vi "数据发送组合-20200825 (子VI).vi"(10 "枚举":T2(ring), 11 "插值后的数组元素":T1) -> (3 "字符串":string)   [LabVIEW 2016, in "数据传输系统-02.lvlib"]
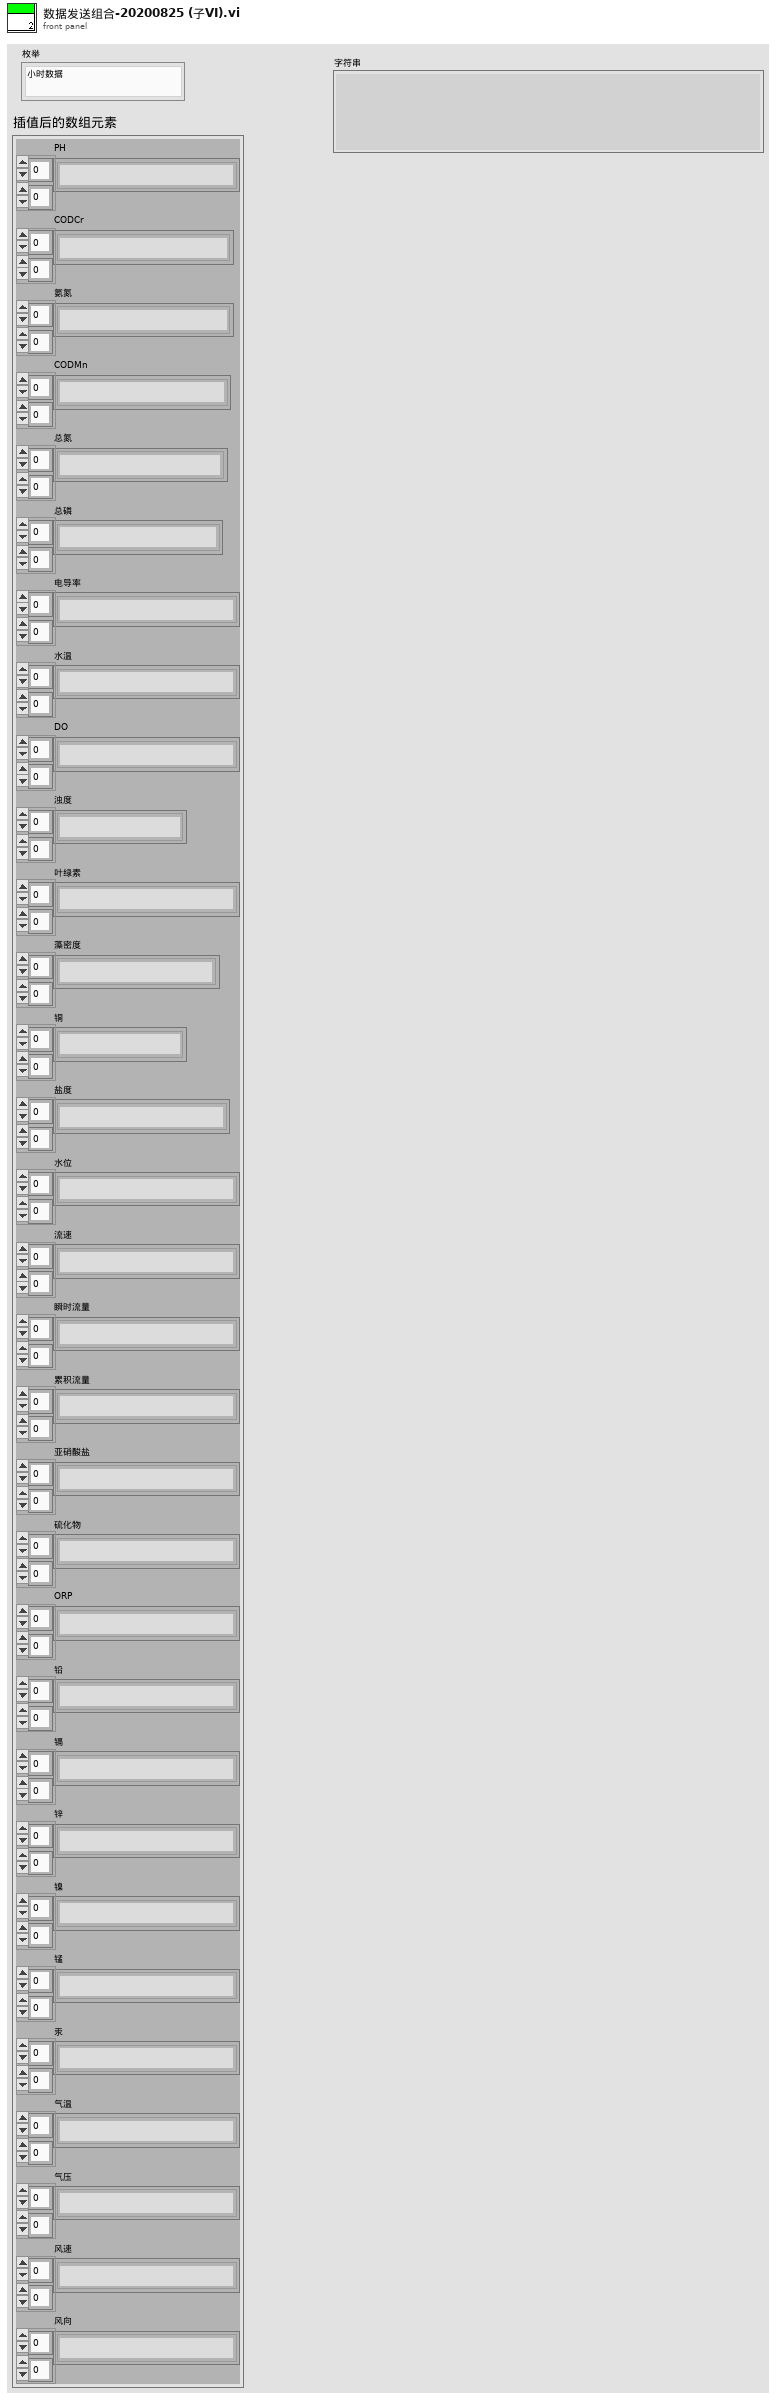
[diagram p1: front panel]
types:
  T1 = cluster{"PH":string[][], "CODCr":string[][], "氨氮":string[][], "CODMn":string[][], "总氮":string[][], "总磷":string[][], "电导率":string[][], "水温":string[][], "DO":string[][], "浊度":string[][], "叶绿素":string[][], "藻密度":string[][], "铜":string[][], "盐度":string[][], "水位":string[][], "流速":string[][], "瞬时流量":string[][], "累积流量":string[][], "亚硝酸盐":string[][], "硫化物":string[][], "ORP":string[][], "铅":string[][], "镉":string[][], "锌":string[][], "镍":string[][], "锰":string[][], "汞":string[][], "气温":string[][], "气压":string[][], "风速":string[][], "风向":string[][]}
  T2 = enum16{"小时数据", "实时数据", "平行样测试", "集成干预测试", "加标回收测试", "核查数据", "空白零点跨度数据", "提取小时数据", "提取实时数据", "操作日志", "仪器参数", "3090仪器参数", "提取仪器参数", "报警信息"}
  T3 = cluster{"CODMn":string, "CODCr":string, "DO":string, "铜":string, "PH":string, "氨氮":string, "比电导率":string, "水温":string, "COD":string, "浊度":string, "总氮":string, "总磷":string, "叶绿素a":string, "藻密度":string, "水位":string, "流速":string, "瞬时流量":string, "累积流量":string, "亚硝酸盐":string, "硫化物":string, "ORP":string, "铅":string, "镉":string, "锌":string, "镍":string, "锰":string, "汞":string, "气温":string, "气压":string, "风速":string, "风向":string}
  T4 = cluster{"CODMn":dbl, "CODCr":dbl, "DO":dbl, "铜":dbl, "PH":dbl, "氨氮":dbl, "比电导率":dbl, "水温":dbl, "COD":dbl, "浊度":dbl, "总氮":dbl, "总磷":dbl, "叶绿素a":dbl, "藻密度":dbl, "水位":dbl, "流速":dbl, "瞬时流量":dbl, "累积流量":dbl, "亚硝酸盐":dbl, "硫化物":dbl, "ORP":dbl, "铅":dbl, "镉":dbl, "锌":dbl, "镍":dbl, "锰":dbl, "汞":dbl, "气温":dbl, "气压":dbl, "风速":dbl, "风向":dbl}
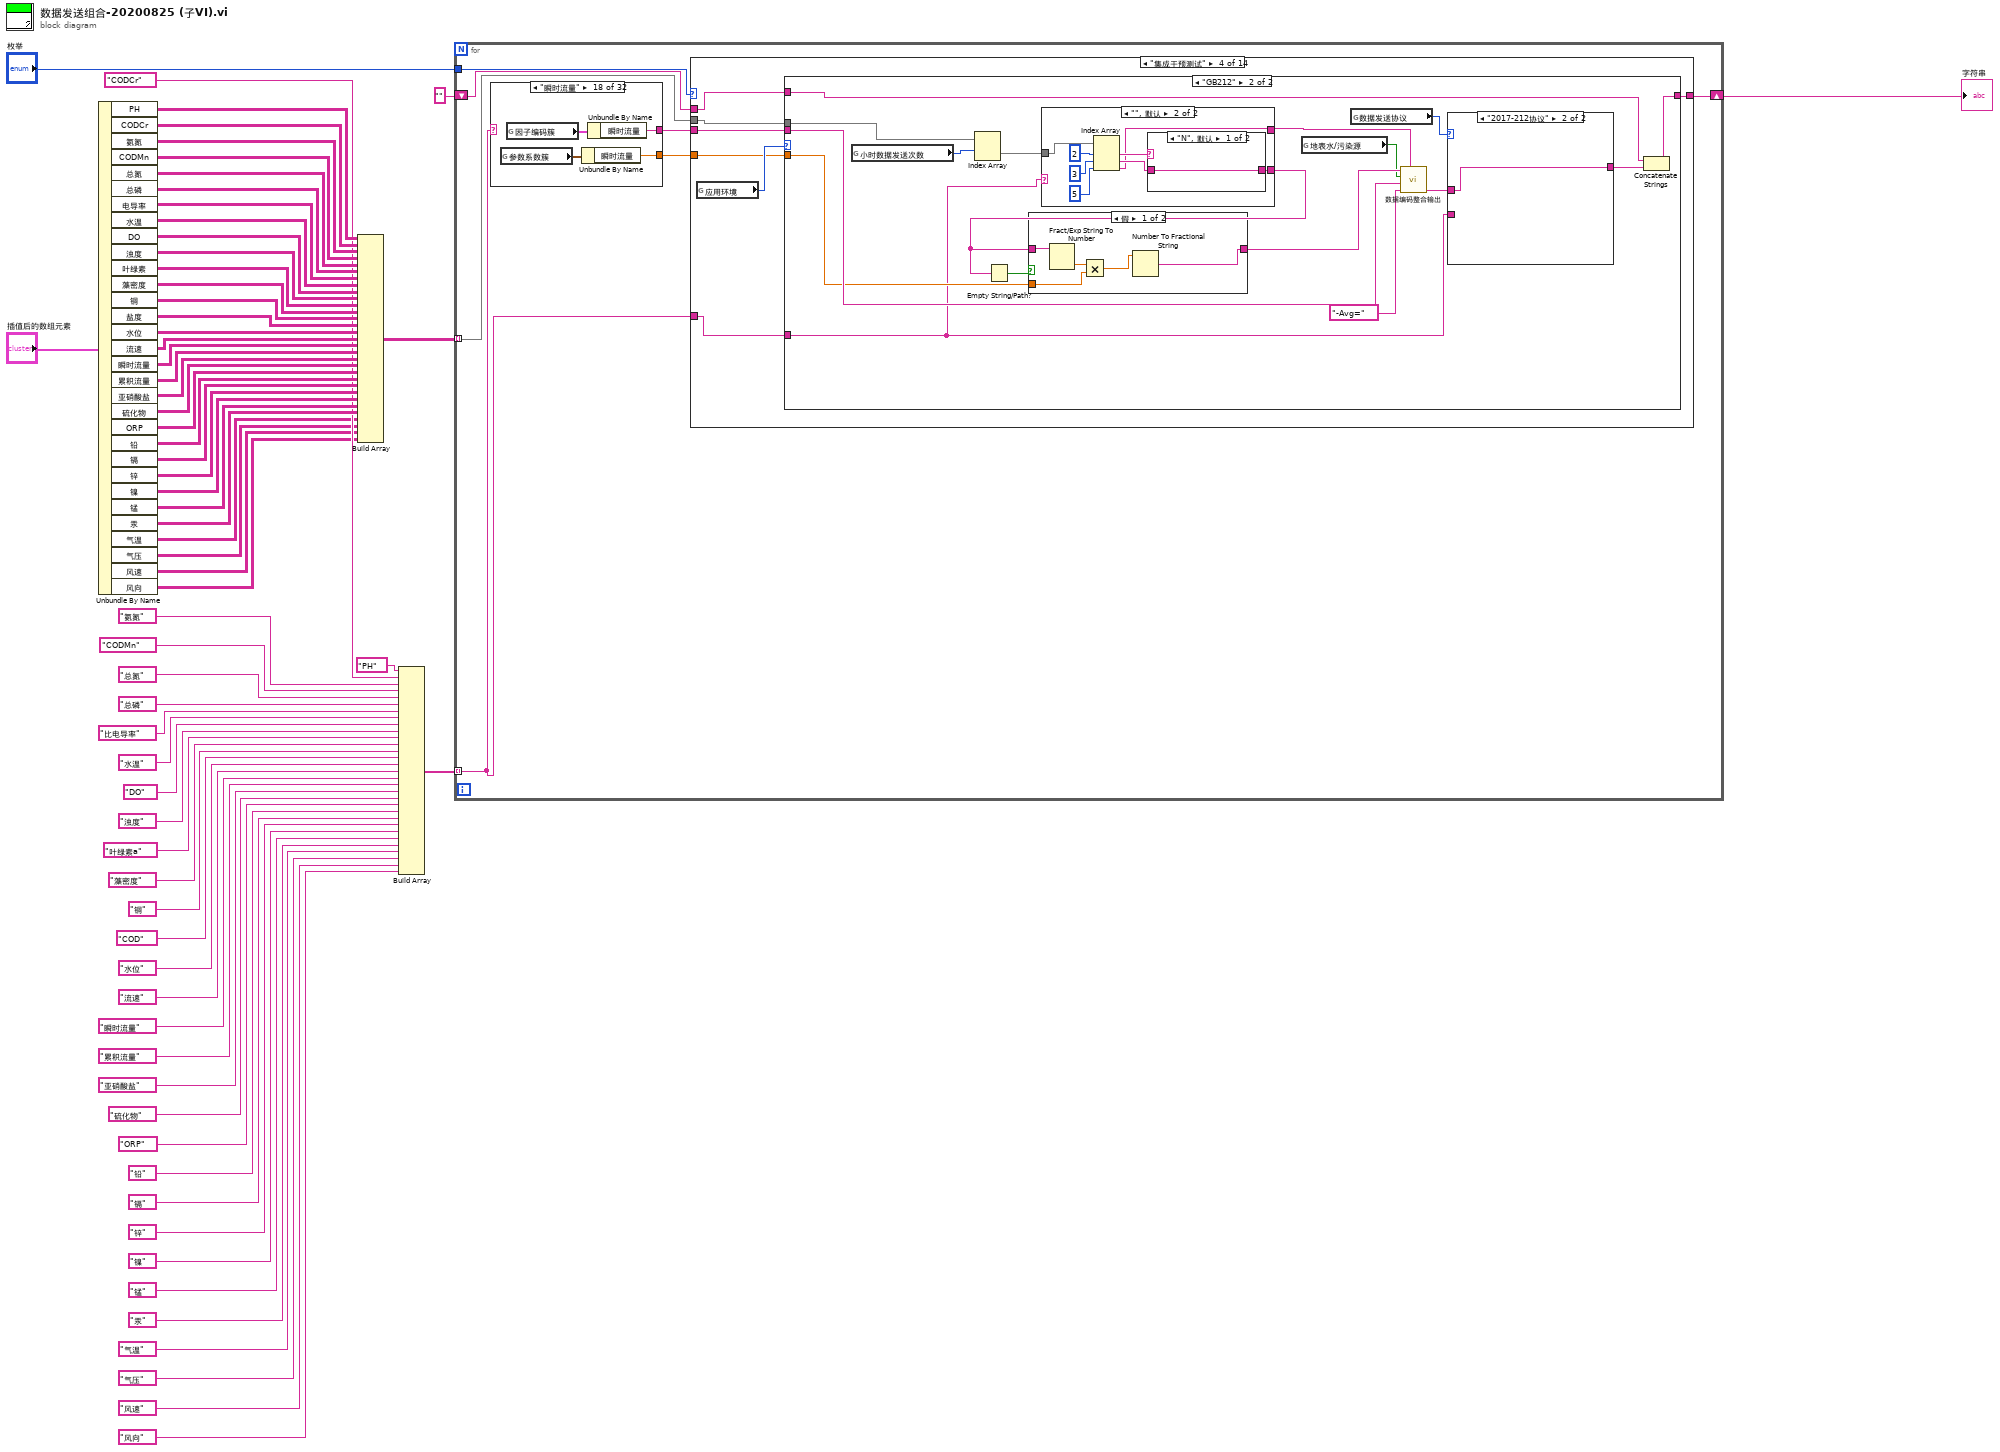
[diagram p0: block diagram]
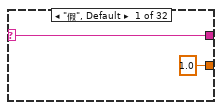
[diagram p2: hidden frame]
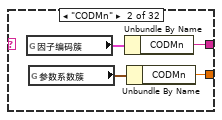
[diagram p3: hidden frame]
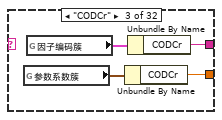
[diagram p4: hidden frame]
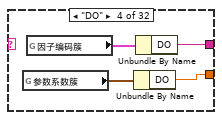
[diagram p5: hidden frame]
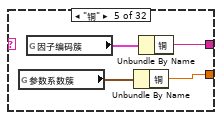
[diagram p6: hidden frame]
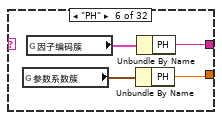
[diagram p7: hidden frame]
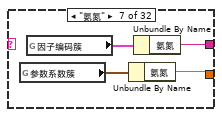
[diagram p8: hidden frame]
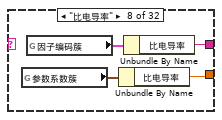
[diagram p9: hidden frame]
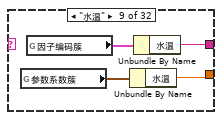
[diagram p10: hidden frame]
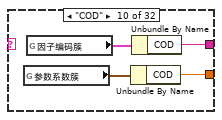
[diagram p11: hidden frame]
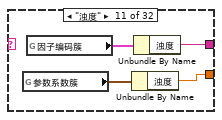
[diagram p12: hidden frame]
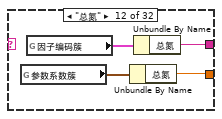
[diagram p13: hidden frame]
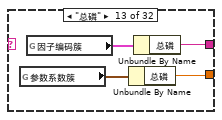
[diagram p14: hidden frame]
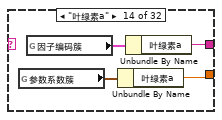
[diagram p15: hidden frame]
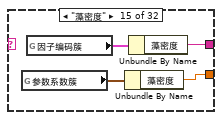
[diagram p16: hidden frame]
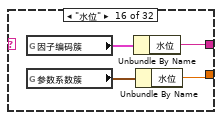
[diagram p17: hidden frame]
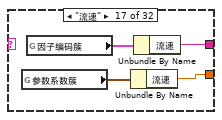
[diagram p18: hidden frame]
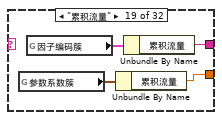
[diagram p19: hidden frame]
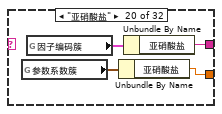
[diagram p20: hidden frame]
diagram:
  n1 = Unbundle By Name("插值后的数组元素") -> ("PH"=w68:string[][], "CODCr"=w67:string[][], "氨氮"=w66:string[][], "CODMn"=w65:string[][], "总氮"=w64:string[][], "总磷"=w63:string[][], "电导率"=w62:string[][], "水温"=w61:string[][], "DO"=w60:string[][], "浊度"=w59:string[][], "叶绿素"=w58:string[][], "藻密度"=w57:string[][], "铜"=w56:string[][], "盐度"=w55:string[][], "水位"=w54:string[][], "流速"=w53:string[][], "瞬时流量"=w52:string[][], "累积流量"=w51:string[][], "亚硝酸盐"=w50:string[][], "硫化物"=w49:string[][], "ORP"=w48:string[][], "铅"=w47:string[][], "镉"=w46:string[][], "锌"=w45:string[][], "镍"=w44:string[][], "锰"=w43:string[][], "汞"=w42:string[][], "气温"=w5:string[][], "气压"=w6:string[][], "风速"=w7:string[][], "风向"=w8:string[][])
  n2 = Build Array(w68, w67, w66, w65, w64, w63, w62, w61, w60, w59, w58, w57, w56, w55, w54, w53, w52, w51, w50, w49, w48, w47, w46, w45, w44, w43, w42, w5, w6, w7, w8) -> (w41:string[][][])
  n3 = Build Array("PH" ("污染物编码"), "CODCr" ("污染物编码"), "氨氮" ("污染物编码"), "CODMn" ("污染物编码"), "总氮" ("污染物编码"), "总磷" ("污染物编码"), "比电导率" ("污染物编码"), "水温" ("污染物编码"), "DO" ("污染物编码"), "浊度" ("污染物编码"), "叶绿素a" ("污染物编码"), "藻密度" ("污染物编码"), "铜" ("污染物编码"), "COD" ("污染物编码"), "水位" ("污染物编码"), "流速" ("污染物编码"), "瞬时流量" ("污染物编码"), "累积流量" ("污染物编码"), "亚硝酸盐" ("污染物编码"), "硫化物" ("污染物编码"), "ORP" ("污染物编码"), "铅" ("污染物编码"), "镉" ("污染物编码"), "锌" ("污染物编码"), "镍" ("污染物编码"), "锰" ("污染物编码"), "汞" ("污染物编码"), "气温" ("污染物编码"), "气压" ("污染物编码"), "风速" ("污染物编码"), "风向" ("污染物编码")) -> (w13:string[])
  n4 = for {
    tunnel: w41 -> [w75] mode=indexing
    tunnel: w13 -> [w70] mode=indexing
    shift-right: [w74] -> w11
    shift-left: "" -> [w73]
    tunnel: "枚举" -> [w72]
    n5 = case shown="\"瞬时流量\"" w70 {
      selector: w70 -> [w77 _ _ _ _ _ _ _ _ _ _ _ _ _ _ _ _ _ _ _ _ _ _ _ _ _ _ _ _ _ _ _]
      tunnel: [w77 w80 w84 w88 w92 w96 w100 w104 w108 w112 w116 w120 w124 w128 w132 w136 w140 w144 w148 w152 w156 w160 w164 w168 w172 w176 w180 w184 w188 w192 w196 w200] -> w71
      tunnel: [1.0 ("风向") w78 w82 w86 w90 w94 w98 w102 w106 w110 w114 w118 w122 w126 w130 w134 w138 w142 w146 w150 w154 w158 w162 w166 w170 w174 w178 w182 w186 w190 w194 w198] -> w69
      frame "假", Default {
      }
      frame "CODMn" {
        n6 = global read "断电保存全局.vi" "因子编码簇"() -> (w81:T3)
        n7 = global read "断电保存全局.vi" "参数系数簇"() -> (w79:T4)
        n8 = Unbundle By Name(w81) -> ("CODMn"=w80:string)
        n9 = Unbundle By Name(w79) -> ("CODMn"=w78:dbl)
      }
      frame "CODCr" {
        n10 = global read "断电保存全局.vi" "参数系数簇"() -> (w83:T4)
        n11 = global read "断电保存全局.vi" "因子编码簇"() -> (w85:T3)
        n12 = Unbundle By Name(w83) -> ("CODCr"=w82:dbl)
        n13 = Unbundle By Name(w85) -> ("CODCr"=w84:string)
      }
      frame "DO" {
        n14 = global read "断电保存全局.vi" "参数系数簇"() -> (w87:T4)
        n15 = global read "断电保存全局.vi" "因子编码簇"() -> (w89:T3)
        n16 = Unbundle By Name(w87) -> ("DO"=w86:dbl)
        n17 = Unbundle By Name(w89) -> ("DO"=w88:string)
      }
      frame "铜" {
        n18 = global read "断电保存全局.vi" "参数系数簇"() -> (w91:T4)
        n19 = global read "断电保存全局.vi" "因子编码簇"() -> (w93:T3)
        n20 = Unbundle By Name(w91) -> ("铜"=w90:dbl)
        n21 = Unbundle By Name(w93) -> ("铜"=w92:string)
      }
      frame "PH" {
        n22 = global read "断电保存全局.vi" "参数系数簇"() -> (w95:T4)
        n23 = global read "断电保存全局.vi" "因子编码簇"() -> (w97:T3)
        n24 = Unbundle By Name(w95) -> ("PH"=w94:dbl)
        n25 = Unbundle By Name(w97) -> ("PH"=w96:string)
      }
      frame "氨氮" {
        n26 = global read "断电保存全局.vi" "参数系数簇"() -> (w99:T4)
        n27 = global read "断电保存全局.vi" "因子编码簇"() -> (w101:T3)
        n28 = Unbundle By Name(w99) -> ("氨氮"=w98:dbl)
        n29 = Unbundle By Name(w101) -> ("氨氮"=w100:string)
      }
      frame "比电导率" {
        n30 = global read "断电保存全局.vi" "参数系数簇"() -> (w103:T4)
        n31 = global read "断电保存全局.vi" "因子编码簇"() -> (w105:T3)
        n32 = Unbundle By Name(w103) -> ("比电导率"=w102:dbl)
        n33 = Unbundle By Name(w105) -> ("比电导率"=w104:string)
      }
      frame "水温" {
        n34 = global read "断电保存全局.vi" "参数系数簇"() -> (w107:T4)
        n35 = global read "断电保存全局.vi" "因子编码簇"() -> (w109:T3)
        n36 = Unbundle By Name(w107) -> ("水温"=w106:dbl)
        n37 = Unbundle By Name(w109) -> ("水温"=w108:string)
      }
      frame "COD" {
        n38 = global read "断电保存全局.vi" "参数系数簇"() -> (w111:T4)
        n39 = global read "断电保存全局.vi" "因子编码簇"() -> (w113:T3)
        n40 = Unbundle By Name(w111) -> ("COD"=w110:dbl)
        n41 = Unbundle By Name(w113) -> ("COD"=w112:string)
      }
      frame "浊度" {
        n42 = global read "断电保存全局.vi" "参数系数簇"() -> (w115:T4)
        n43 = global read "断电保存全局.vi" "因子编码簇"() -> (w117:T3)
        n44 = Unbundle By Name(w115) -> ("浊度"=w114:dbl)
        n45 = Unbundle By Name(w117) -> ("浊度"=w116:string)
      }
      frame "总氮" {
        n46 = global read "断电保存全局.vi" "参数系数簇"() -> (w119:T4)
        n47 = global read "断电保存全局.vi" "因子编码簇"() -> (w121:T3)
        n48 = Unbundle By Name(w119) -> ("总氮"=w118:dbl)
        n49 = Unbundle By Name(w121) -> ("总氮"=w120:string)
      }
      frame "总磷" {
        n50 = global read "断电保存全局.vi" "参数系数簇"() -> (w123:T4)
        n51 = global read "断电保存全局.vi" "因子编码簇"() -> (w125:T3)
        n52 = Unbundle By Name(w123) -> ("总磷"=w122:dbl)
        n53 = Unbundle By Name(w125) -> ("总磷"=w124:string)
      }
      frame "叶绿素a" {
        n54 = global read "断电保存全局.vi" "参数系数簇"() -> (w127:T4)
        n55 = global read "断电保存全局.vi" "因子编码簇"() -> (w129:T3)
        n56 = Unbundle By Name(w127) -> ("叶绿素a"=w126:dbl)
        n57 = Unbundle By Name(w129) -> ("叶绿素a"=w128:string)
      }
      frame "藻密度" {
        n58 = global read "断电保存全局.vi" "参数系数簇"() -> (w131:T4)
        n59 = global read "断电保存全局.vi" "因子编码簇"() -> (w133:T3)
        n60 = Unbundle By Name(w131) -> ("藻密度"=w130:dbl)
        n61 = Unbundle By Name(w133) -> ("藻密度"=w132:string)
      }
      frame "水位" {
        n62 = global read "断电保存全局.vi" "因子编码簇"() -> (w137:T3)
        n63 = global read "断电保存全局.vi" "参数系数簇"() -> (w135:T4)
        n64 = Unbundle By Name(w137) -> ("水位"=w136:string)
        n65 = Unbundle By Name(w135) -> ("水位"=w134:dbl)
      }
      frame "流速" {
        n66 = global read "断电保存全局.vi" "参数系数簇"() -> (w139:T4)
        n67 = global read "断电保存全局.vi" "因子编码簇"() -> (w141:T3)
        n68 = Unbundle By Name(w139) -> ("流速"=w138:dbl)
        n69 = Unbundle By Name(w141) -> ("流速"=w140:string)
      }
      frame "瞬时流量" {
        n70 = global read "断电保存全局.vi" "参数系数簇"() -> (w143:T4)
        n71 = global read "断电保存全局.vi" "因子编码簇"() -> (w145:T3)
        n72 = Unbundle By Name(w143) -> ("瞬时流量"=w142:dbl)
        n73 = Unbundle By Name(w145) -> ("瞬时流量"=w144:string)
      }
      frame "累积流量" {
        n74 = global read "断电保存全局.vi" "参数系数簇"() -> (w147:T4)
        n75 = global read "断电保存全局.vi" "因子编码簇"() -> (w149:T3)
        n76 = Unbundle By Name(w147) -> ("累积流量"=w146:dbl)
        n77 = Unbundle By Name(w149) -> ("累积流量"=w148:string)
      }
      frame "亚硝酸盐" {
        n78 = global read "断电保存全局.vi" "参数系数簇"() -> (w151:T4)
        n79 = global read "断电保存全局.vi" "因子编码簇"() -> (w153:T3)
        n80 = Unbundle By Name(w151) -> ("亚硝酸盐"=w150:dbl)
        n81 = Unbundle By Name(w153) -> ("亚硝酸盐"=w152:string)
      }
      frame "硫化物" {
        n82 = global read "断电保存全局.vi" "参数系数簇"() -> (w155:T4)
        n83 = global read "断电保存全局.vi" "因子编码簇"() -> (w157:T3)
        n84 = Unbundle By Name(w155) -> ("硫化物"=w154:dbl)
        n85 = Unbundle By Name(w157) -> ("硫化物"=w156:string)
      }
      frame "ORP" {
        n86 = global read "断电保存全局.vi" "参数系数簇"() -> (w159:T4)
        n87 = global read "断电保存全局.vi" "因子编码簇"() -> (w161:T3)
        n88 = Unbundle By Name(w159) -> ("ORP"=w158:dbl)
        n89 = Unbundle By Name(w161) -> ("ORP"=w160:string)
      }
      frame "铅" {
        n90 = global read "断电保存全局.vi" "参数系数簇"() -> (w163:T4)
        n91 = global read "断电保存全局.vi" "因子编码簇"() -> (w165:T3)
        n92 = Unbundle By Name(w165) -> ("铅"=w164:string)
        n93 = Unbundle By Name(w163) -> ("铅"=w162:dbl)
      }
      frame "镉" {
        n94 = global read "断电保存全局.vi" "参数系数簇"() -> (w167:T4)
        n95 = global read "断电保存全局.vi" "因子编码簇"() -> (w169:T3)
        n96 = Unbundle By Name(w167) -> ("镉"=w166:dbl)
        n97 = Unbundle By Name(w169) -> ("镉"=w168:string)
      }
      frame "锌" {
        n98 = global read "断电保存全局.vi" "参数系数簇"() -> (w171:T4)
        n99 = global read "断电保存全局.vi" "因子编码簇"() -> (w173:T3)
        n100 = Unbundle By Name(w171) -> ("锌"=w170:dbl)
        n101 = Unbundle By Name(w173) -> ("锌"=w172:string)
      }
      frame "镍" {
        n102 = global read "断电保存全局.vi" "参数系数簇"() -> (w175:T4)
        n103 = global read "断电保存全局.vi" "因子编码簇"() -> (w177:T3)
        n104 = Unbundle By Name(w175) -> ("镍"=w174:dbl)
        n105 = Unbundle By Name(w177) -> ("镍"=w176:string)
      }
      frame "锰" {
        n106 = global read "断电保存全局.vi" "参数系数簇"() -> (w179:T4)
        n107 = global read "断电保存全局.vi" "因子编码簇"() -> (w181:T3)
        n108 = Unbundle By Name(w181) -> ("锰"=w180:string)
        n109 = Unbundle By Name(w179) -> ("锰"=w178:dbl)
      }
      frame "汞" {
        n110 = global read "断电保存全局.vi" "参数系数簇"() -> (w183:T4)
        n111 = global read "断电保存全局.vi" "因子编码簇"() -> (w185:T3)
        n112 = Unbundle By Name(w185) -> ("汞"=w184:string)
        n113 = Unbundle By Name(w183) -> ("汞"=w182:dbl)
      }
      frame "气温" {
        n114 = global read "断电保存全局.vi" "因子编码簇"() -> (w189:T3)
        n115 = global read "断电保存全局.vi" "参数系数簇"() -> (w187:T4)
        n116 = Unbundle By Name(w189) -> ("气温"=w188:string)
        n117 = Unbundle By Name(w187) -> ("气温"=w186:dbl)
      }
      frame "气压" {
        n118 = global read "断电保存全局.vi" "参数系数簇"() -> (w191:T4)
        n119 = global read "断电保存全局.vi" "因子编码簇"() -> (w193:T3)
        n120 = Unbundle By Name(w191) -> ("气压"=w190:dbl)
        n121 = Unbundle By Name(w193) -> ("气压"=w192:string)
      }
      frame "风速" {
        n122 = global read "断电保存全局.vi" "参数系数簇"() -> (w195:T4)
        n123 = global read "断电保存全局.vi" "因子编码簇"() -> (w197:T3)
        n124 = Unbundle By Name(w195) -> ("风速"=w194:dbl)
        n125 = Unbundle By Name(w197) -> ("风速"=w196:string)
      }
      frame "风向" {
        n126 = global read "断电保存全局.vi" "参数系数簇"() -> (w199:T4)
        n127 = global read "断电保存全局.vi" "因子编码簇"() -> (w201:T3)
        n128 = Unbundle By Name(w201) -> ("风向"=w200:string)
        n129 = Unbundle By Name(w199) -> ("风向"=w198:dbl)
      }
    }
    n130 = case shown="\"集成干预测试\"" w72 {
      tunnel: w75 -> [w214 w258 w289 w298 w352 w359 w369 w392 w413 w450 w467 w472 w482 w502]
      tunnel: w71 -> [w210 w251 w288 w299 w353 w358 w368 w386 w412 w438 w464 w470 w481 w505]
      tunnel: [w213 w255 w290 w296 w354 w355 w365 w383 w411 w445 w461 w469 w477 w490] -> w74
      tunnel: w73 -> [w212 w256 w292 w297 w349 w357 w366 w384 w414 w446 w462 w471 w478 w485]
      tunnel: w70 -> [w207 w250 _ w293 _ _ _ _ _ _ _ _ _ w500]
      tunnel: w69 -> [w204 w246 _ w294 _ _ _ w379 w407 _ _ _ _ _]
      frame "小时数据", Default {
        n131 = global read "全局 小时数据发送次数.vi" "小时数据发送次数"() -> (w218:i32)
        n132 = Index Array(array=w214, index (row)=w218) -> (element=w217:string[])  [unwired: 1 in]
        n133 = case shown="\"风速\", \"风向\", \"累积流量\", \"流速\", \"气温\", \"气压\", \"水位\", \"瞬时流量\"" w207 {
          tunnel: w217 -> [w228 w231]
          tunnel: [w225 w230] -> w205
          tunnel: ["N" ("字符串") w229] -> w215
          frame "风速", "风向", "累积流量", "流速", "气温", "气压", "水位", "瞬时流量" {
            n134 = Index Array(array=w228, index=1 ("索引")) -> (element=w225:string)
          }
          frame "", Default {
            n135 = Index Array(array=w231, index #1=2 ("索引"), index #2=3 ("索引"), index #3=5 ("索引")) -> (element #1=w234:string, element #2=w233:string, element #3=w229:string)
            n136 = case shown="\"N\", 默认" w234 {
              tunnel: [w237 ""] -> w230
              tunnel: w233 -> [w237 _]
              frame "N", Default {
              }
              frame "M" {
              }
            }
          }
        }
        n137 = Empty String/Path?(string/path=w205) -> (empty?=w206:bool)
        n138 = case shown="假" w206 {
          tunnel: w205 -> [w222 w224]
          tunnel: w204 -> [w221 _]
          tunnel: [w219 w224] -> w203
          frame False {
            n139 = Fract/Exp String To Number(string=w222) -> (number=w223:dbl)  [unwired: 3 in, 1 out]
            n140 = Multiply(x=w223, y=w221) -> (x*y=w220:dbl)
            n141 = Number To Fractional String(number=w220) -> (F-format string=w219:string)  [unwired: 3 in]
          }
          frame True {
            # "空"
          }
        }
        n142 = global read "断电保存全局.vi" "地表水/污染源"() -> (w202:bool)
        n143 = global read "断电保存全局.vi" "数据发送协议"() -> (w211:enum16{"2005-212协议", "2017-212协议"})
        n144 = call "数据编码整合输出.vi"("数据标识"=w215, "数据类型"="-Avg=", "污染物编码"=w210, "地表水/污染源"=w202, "数据值"=w203) -> ("编码输出"=w209:string)  [unwired: 6 in]
        n145 = case shown="\"2017-212协议\"" w211 {
          tunnel: w207 -> [w241 _]
          tunnel: w209 -> [w239 w244]
          tunnel: [w240 w244] -> w208
          frame "2005-212协议", Default {
            n146 = case shown="\"风速\", \"风向\", \"累积流量\", \"流速\", \"气温\", \"气压\", \"水位\"" w241 {
              tunnel: [w242 ""] -> w240
              tunnel: w239 -> [w242 _]
              frame "假", Default {
              }
              frame "风速", "风向", "累积流量", "流速", "气温", "气压", "水位" {
              }
            }
          }
          frame "2017-212协议" {
          }
        }
        n147 = Concatenate Strings(w212, w208) -> (w213:string)
      }
      frame "实时数据" {
        n148 = global read "全局 小时数据发送次数.vi" "小时数据发送次数"() -> (w259:i32)
        n149 = Index Array(array=w258, index (row)=w259) -> (element=w260:string[])  [unwired: 1 in]
        n150 = case shown="\"\", 默认" w250 {
          tunnel: w260 -> [w269 w273 w279]
          tunnel: [w268 w272 w278] -> w248
          tunnel: ["N" ("字符串") "N" ("字符串") w276] -> w257
          frame "累积流量", "流速", "水位", "瞬时流量" {
            n151 = Index Array(array=w269, index=1 ("索引")) -> (element=w268:string)
          }
          frame "风速", "风向", "气温", "气压" {
            n152 = Index Array(array=w273, index=1 ("索引")) -> (element=w272:string)
          }
          frame "", Default {
            n153 = Index Array(array=w279, index #1=3 ("索引"), index #2=5 ("索引")) -> (element #1=w278:string, element #2=w276:string)
          }
        }
        n154 = Empty String/Path?(string/path=w248) -> (empty?=w249:bool)
        n155 = case shown="假" w249 {
          tunnel: w248 -> [w265 w267]
          tunnel: w246 -> [w264 _]
          tunnel: [w262 w267] -> w247
          frame False {
            n156 = Fract/Exp String To Number(string=w265) -> (number=w266:dbl)  [unwired: 3 in, 1 out]
            n157 = Multiply(x=w266, y=w264) -> (x*y=w263:dbl)
            n158 = Number To Fractional String(number=w263) -> (F-format string=w262:string)  [unwired: 3 in]
          }
          frame True {
            # "空"
          }
        }
        n159 = global read "断电保存全局.vi" "数据发送协议"() -> (w254:enum16{"2005-212协议", "2017-212协议"})
        n160 = call "数据编码整合输出.vi"("数据标识"=w257, "数据类型"="-Rtd=", "污染物编码"=w251, "地表水/污染源"=FALSE, "数据值"=w247) -> ("编码输出"=w253:string)  [unwired: 6 in]
        n161 = case shown="\"2017-212协议\"" w254 {
          tunnel: w250 -> [w283 _]
          tunnel: w253 -> [w281 w286]
          tunnel: [w282 w286] -> w252
          frame "2005-212协议", Default {
            n162 = case shown="\"假\", 默认" w283 {
              tunnel: [w284 ""] -> w282
              tunnel: w281 -> [w284 _]
              frame "假", Default {
              }
              frame "风速", "风向", "累积流量", "流速", "气温", "气压", "水位" {
              }
            }
          }
          frame "2017-212协议" {
          }
        }
        n163 = Concatenate Strings(w256, w252) -> (w255:string)
      }
      frame "平行样测试" {
        n164 = global read "全局 小时数据发送次数.vi" "小时数据发送次数"() -> (w287:i32)
        n165 = call "平行样集成干预数据组合(子VI).vi"("污染物编码"=w288, "数据输入"=w289, "小时数据发送次数"=w287) -> ("输出组合"=w291:string)  [unwired: 8 in]
        n166 = Concatenate Strings(w292, w291) -> (w290:string)
      }
      frame "集成干预测试" {
        n167 = global read "断电保存全局.vi" "应用环境"() -> (w295:enum16{"STD", "GB212"})
        n168 = case shown="\"GB212\"" w295 {
          tunnel: w299 -> [w303 w309]
          tunnel: w298 -> [w302 w310]
          tunnel: w297 -> [w301 w311]
          tunnel: [w300 w306] -> w296
          tunnel: w294 -> [_ w308]
          tunnel: w293 -> [_ w307]
          frame "STD", Default {
            n169 = global read "全局 小时数据发送次数.vi" "小时数据发送次数"() -> (w304:i32)
            n170 = call "平行样集成干预数据组合(子VI).vi"("污染物编码"=w303, "数据输入"=w302, "小时数据发送次数"=w304) -> ("输出组合"=w305:string)  [unwired: 8 in]
            n171 = Concatenate Strings(w301, w305) -> (w300:string)
          }
          frame "GB212" {
            n172 = global read "全局 小时数据发送次数.vi" "小时数据发送次数"() -> (w322:i32)
            n173 = Index Array(array=w310, index (row)=w322) -> (element=w321:string[])  [unwired: 1 in]
            n174 = case shown="\"\", 默认" w307 {
              tunnel: w321 -> [w332 w335]
              tunnel: [w329 w334] -> w314
              tunnel: ["N" ("字符串") w333] -> w319
              frame "风速", "风向", "累积流量", "流速", "气温", "气压", "水位", "瞬时流量" {
                n175 = Index Array(array=w332, index=1 ("索引")) -> (element=w329:string)
              }
              frame "", Default {
                n176 = Index Array(array=w335, index #1=2 ("索引"), index #2=3 ("索引"), index #3=5 ("索引")) -> (element #1=w338:string, element #2=w337:string, element #3=w333:string)
                n177 = case shown="\"N\", 默认" w338 {
                  tunnel: [w341 ""] -> w334
                  tunnel: w337 -> [w341 _]
                  frame "N", Default {
                  }
                  frame "M" {
                  }
                }
              }
            }
            n178 = Empty String/Path?(string/path=w314) -> (empty?=w315:bool)
            n179 = case shown="假" w315 {
              tunnel: w314 -> [w326 w328]
              tunnel: w308 -> [w325 _]
              tunnel: [w323 w328] -> w313
              frame False {
                n180 = Fract/Exp String To Number(string=w326) -> (number=w327:dbl)  [unwired: 3 in, 1 out]
                n181 = Multiply(x=w327, y=w325) -> (x*y=w324:dbl)
                n182 = Number To Fractional String(number=w324) -> (F-format string=w323:string)  [unwired: 3 in]
              }
              frame True {
                # "空"
              }
            }
            n183 = global read "断电保存全局.vi" "地表水/污染源"() -> (w312:bool)
            n184 = global read "断电保存全局.vi" "数据发送协议"() -> (w318:enum16{"2005-212协议", "2017-212协议"})
            n185 = call "数据编码整合输出.vi"("数据标识"=w319, "数据类型"="-Avg=", "污染物编码"=w309, "地表水/污染源"=w312, "数据值"=w313) -> ("编码输出"=w317:string)  [unwired: 6 in]
            n186 = case shown="\"2017-212协议\"" w318 {
              tunnel: w307 -> [w345 _]
              tunnel: w317 -> [w343 w348]
              tunnel: [w344 w348] -> w316
              frame "2005-212协议", Default {
                n187 = case shown="\"假\", 默认" w345 {
                  tunnel: [w346 ""] -> w344
                  tunnel: w343 -> [w346 _]
                  frame "假", Default {
                  }
                  frame "风速", "风向", "累积流量", "流速", "气温", "气压", "水位" {
                  }
                }
              }
              frame "2017-212协议" {
              }
            }
            n188 = Concatenate Strings(w311, w316) -> (w306:string)
          }
        }
      }
      frame "加标回收测试" {
        n189 = global read "全局 小时数据发送次数.vi" "小时数据发送次数"() -> (w351:i32)
        n190 = call "加标回收数据组合 (子VI).vi"("小时数据发送次数"=w351, "数据"=w352, "污染物编码"=w353) -> ("组合输出"=w350:string)  [unwired: 7 in, 1 out]
        n191 = Concatenate Strings(w349, w350) -> (w354:string)
      }
      frame "核查数据" {
        n192 = global read "全局 小时数据发送次数.vi" "小时数据发送次数"() -> (w360:i32)
        n193 = call "标样核查数据组合(子VI).vi"("小时数据发送次数"=w360, "数据输入"=w359, "污染物编码"=w358) -> ("输出组合"=w356:string)  [unwired: 8 in]
        n194 = Concatenate Strings(w357, w356) -> (w355:string)
      }
      frame "空白零点跨度数据" {
        n195 = global read "全局 小时数据发送次数.vi" "小时数据发送次数"() -> (w371:i32)
        n196 = Index Array(array=w369, index (row)=w371) -> (element=w375:string[])  [unwired: 1 in]
        n197 = Index Array(array=w375, index #1=0 ("索引"), index #2=3 ("索引"), index #3=7 ("索引"), index #4=8 ("索引")) -> (element #2=w370:string, element #3=w372:string, element #4=w361:string)  [unwired: 1 out]
        n198 = Empty String/Path?(string/path=w361) -> (empty?=w363:bool)
        n199 = case shown="真" w363 {
          tunnel: [w377 "0" ("span value")] -> w362
          tunnel: w361 -> [w377 _]
          frame False {
          }
          frame True {
          }
        }
        n200 = call "零点跨度数据组合 (子VI).vi"("span value"=w362, "standard value"=w372, "check value"=w370, "污染物编码"=w368) -> ("组合输出"=w367:string)  [unwired: 7 in]
        n201 = Concatenate Strings(w366, w367) -> (w365:string)
      }
      frame "提取小时数据" {
        n202 = global read "全局 小时数据发送次数.vi" "小时数据发送次数"() -> (w393:i32)
        n203 = Index Array(array=w392, index (row)=w393) -> (element=w391:string[])  [unwired: 1 in]
        n204 = Index Array(array=w391, index #2=1 ("索引")) -> (element #2=w380:string)  [unwired: 1 in, 1 out]
        n205 = Empty String/Path?(string/path=w380) -> (empty?=w382:bool)
        n206 = case shown="假" w382 {
          tunnel: w380 -> [w398 w400]
          tunnel: w379 -> [w397 _]
          tunnel: [w395 w400] -> w381
          frame False {
            n207 = Fract/Exp String To Number(string=w398) -> (number=w399:dbl)  [unwired: 3 in, 1 out]
            n208 = Multiply(x=w399, y=w397) -> (x*y=w396:dbl)
            n209 = Number To Fractional String(number=w396) -> (F-format string=w395:string)  [unwired: 3 in]
          }
          frame True {
            # "空"
          }
        }
        n210 = global read "断电保存全局.vi" "数据发送协议"() -> (w388:enum16{"2005-212协议", "2017-212协议"})
        n211 = call "数据编码整合输出.vi"("数据标识"="N", "数据类型"="-Avg=", "污染物编码"=w386, "数据值"=w381) -> ("编码输出"=w385:string)  [unwired: 7 in]
        n212 = case shown="\"2005-212协议\", 默认" w388 {
          tunnel: w386 -> [w403 _]
          tunnel: w385 -> [w401 w406]
          tunnel: [w402 w406] -> w387
          frame "2005-212协议", Default {
            n213 = case shown="\"假\", 默认" w403 {
              tunnel: [w404 ""] -> w402
              tunnel: w401 -> [w404 _]
              frame "假", Default {
              }
              frame "累积流量", "流速", "水位" {
              }
            }
          }
          frame "2017-212协议" {
          }
        }
        n214 = Concatenate Strings(w384, w387) -> (w383:string)
      }
      frame "提取实时数据" {
        n215 = global read "全局 小时数据发送次数.vi" "小时数据发送次数"() -> (w420:i32)
        n216 = Index Array(array=w413, index (row)=w420) -> (element=w421:string[])  [unwired: 1 in]
        n217 = Index Array(array=w421, index #1=3 ("索引"), index #2=5 ("索引")) -> (element #1=w408:string, element #2=w418:string)
        n218 = Empty String/Path?(string/path=w408) -> (empty?=w410:bool)
        n219 = case shown="假" w410 {
          tunnel: w408 -> [w427 w429]
          tunnel: w407 -> [w426 _]
          tunnel: [w424 w429] -> w409
          frame False {
            n220 = Fract/Exp String To Number(string=w427) -> (number=w428:dbl)  [unwired: 3 in, 1 out]
            n221 = Multiply(x=w428, y=w426) -> (x*y=w425:dbl)
            n222 = Number To Fractional String(number=w425) -> (F-format string=w424:string)  [unwired: 3 in]
          }
          frame True {
            # "空"
          }
        }
        n223 = global read "断电保存全局.vi" "数据发送协议"() -> (w417:enum16{"2005-212协议", "2017-212协议"})
        n224 = call "数据编码整合输出.vi"("数据标识"=w418, "数据类型"="-Rtd=", "污染物编码"=w412, "数据值"=w409) -> ("编码输出"=w416:string)  [unwired: 7 in]
        n225 = case shown="\"2017-212协议\"" w417 {
          tunnel: w412 -> [w432 _]
          tunnel: w416 -> [w430 w435]
          tunnel: [w431 w435] -> w415
          frame "2005-212协议", Default {
            n226 = case shown="\"累积流量\", \"流速\", \"水位\"" w432 {
              tunnel: [w433 ""] -> w431
              tunnel: w430 -> [w433 _]
              frame "假", Default {
              }
              frame "累积流量", "流速", "水位" {
              }
            }
          }
          frame "2017-212协议" {
          }
        }
        n227 = Concatenate Strings(w414, w415) -> (w411:string)
      }
      frame "操作日志" {
        n228 = global read "断电保存全局.vi" "因子编码簇"() -> (w441:T3)
        n229 = global read "全局 小时数据发送次数.vi" "小时数据发送次数"() -> (w454:i32)
        n230 = Unbundle By Name(w441) -> ("DO"=w440:string)
        n231 = Equal?(x=w438, y=w440) -> (x = y?=w436:bool)
        n232 = Index Array(array=w450, index (row)=w454) -> (element=w449:string[])  [unwired: 1 in]
        n233 = Index Array(array=w449, index #1=0 ("索引"), index #2=2 ("索引")) -> (element #2=w448:string)  [unwired: 1 out]
        n234 = Empty String/Path?(string/path=w448) -> (empty?=w453:bool)
        n235 = Select(t="w00000", s=w436, f=w438) -> (s? t:f=w437:string)
        n236 = Select(t="i21001", s=w436, f="i11001") -> (s? t:f=w442:string)
        n237 = case shown="假" w453 {
          tunnel: [w458 ""] -> w447
          tunnel: w448 -> [w456 _]
          tunnel: w437 -> [w457 _]
          tunnel: w442 -> [w455 _]
          frame False {
            n238 = Format Into String(format string="PolId=%s,%s-Info=//%s//;" ("格式字符串"), w457, w455, w456) -> (resulting string=w458:string)  [unwired: 2 in, 1 out]
          }
          frame True {
          }
        }
        n239 = Concatenate Strings(w446, w447) -> (w445:string)
      }
      frame "仪器参数" {
        n240 = global read "全局 小时数据发送次数.vi" "小时数据发送次数"() -> (w468:i32)
        n241 = Index Array(array=w467, index (row)=w468) -> (element=w465:string[])  [unwired: 1 in]
        n242 = call "关键参数组合 (子VI).vi"("table"="仪器参数", "因子编码"=w464, "DO"=w465) -> ("字符串"=w463:string)  [unwired: 8 in]
        n243 = Concatenate Strings(w462, w463) -> (w461:string)
      }
      frame "3090仪器参数" {
        n244 = global read "全局 小时数据发送次数.vi" "小时数据发送次数"() -> (w476:i32)
        n245 = Index Array(array=w472, index (row)=w476) -> (element=w474:string[])  [unwired: 1 in]
        n246 = call "关键参数组合 (子VI).vi"("table"="3090仪器参数", "因子编码"=w470, "DO"=w474) -> ("字符串"=w473:string)  [unwired: 8 in]
        n247 = Concatenate Strings(w471, w473) -> (w469:string)
      }
      frame "提取仪器参数" {
        n248 = global read "全局 小时数据发送次数.vi" "小时数据发送次数"() -> (w483:i32)
        n249 = Index Array(array=w482, index (row)=w483) -> (element=w480:string[])  [unwired: 1 in]
        n250 = call "提取仪器参数 (子VI).vi"("因子编码"=w481, "数据输入"=w480) -> ("字符串"=w479:string)  [unwired: 9 in]
        n251 = Concatenate Strings(w478, w479) -> (w477:string)
      }
      frame "报警信息" {
        n252 = case shown="\"CODCr\"" w500 {
          tunnel: [u16 0 ("register") w522 w525 w528 w531 w534] -> w498
          frame "假", Default {
          }
          frame "CODMn" {
            n253 = global read "全局1.vi" "register values"() -> (w524:u16[])
            n254 = Index Array(array=w524, index=1 ("索引")) -> (element=w522:u16)
          }
          frame "氨氮" {
            n255 = global read "全局1.vi" "register values"() -> (w527:u16[])
            n256 = Index Array(array=w527, index=2 ("索引")) -> (element=w525:u16)
          }
          frame "总磷" {
            n257 = global read "全局1.vi" "register values"() -> (w530:u16[])
            n258 = Index Array(array=w530, index=3 ("索引")) -> (element=w528:u16)
          }
          frame "总氮" {
            n259 = global read "全局1.vi" "register values"() -> (w533:u16[])
            n260 = Index Array(array=w533, index=4 ("索引")) -> (element=w531:u16)
          }
          frame "CODCr" {
            n261 = global read "全局1.vi" "register values"() -> (w536:u16[])
            n262 = Index Array(array=w536, index=5 ("索引")) -> (element=w534:u16)
          }
        }
        n263 = global read "断电保存全局.vi" "因子编码簇"() -> (w508:T3)
        n264 = global read "全局 小时数据发送次数.vi" "小时数据发送次数"() -> (w503:i32)
        n265 = Unbundle By Name(w508) -> ("DO"=w507:string)
        n266 = Equal?(x=w505, y=w507) -> (x = y?=w495:bool)
        n267 = Index Array(array=w502, index (row)=w503) -> (element=w501:string[])  [unwired: 1 in]
        n268 = Select(t="w00000", s=w495, f=w505) -> (s? t:f=w504:string)
        n269 = Index Array(array=w501, index #1=0 ("索引"), index #2=2 ("索引")) -> (element #1=w492:string, element #2=w514:string)
        n270 = Empty String/Path?(string/path=w514) -> (empty?=w513:bool)
        n271 = Number To Decimal String(number=w498) -> (decimal integer string=w499:string)  [unwired: 1 in]
        n272 = Select(t="i22001", s=w495, f="i12001") -> (s? t:f=w494:string)
        n273 = Select(t="i22003", s=w495, f="i12031") -> (s? t:f=w493:string)
        n274 = case shown="假" w513 {
          tunnel: [w544 ""] -> w489
          tunnel: w514 -> [w538 _]
          tunnel: w504 -> [w541 _]
          tunnel: w499 -> [w542 _]
          tunnel: w494 -> [w540 _]
          tunnel: w493 -> [w539 _]
          frame False {
            n275 = call "告警信息文本转换为协议i12031值.vi"("字符串"=w538) -> ("十进制整型字符串"=w537:string)  [unwired: 10 in]
            n276 = Format Into String(format string="PolId=%s,%s-Info=%s,i12002-Info=0,i12003-Info=100,%s-Info=%s;" ("格式字符串"), w541, w540, w542, w539, w537) -> (resulting string=w544:string)  [unwired: 2 in, 1 out]
          }
          frame True {
          }
        }
        n277 = Empty String/Path?(string/path=w489) -> (empty?=w488:bool)
        n278 = Empty String/Path?(string/path=w485) -> (empty?=w484:bool)
        n279 = Not(x=w488) -> (.not. x?=w487:bool)
        n280 = And(x=w484, y=w487) -> (x .and. y?=w486:bool)
        n281 = Concatenate Strings(w485, w489) -> (w491:string)
        n282 = case shown="真" w486 {
          tunnel: w492 -> [_ w518]
          tunnel: w491 -> [w515 w517]
          tunnel: [w515 w516] -> w490
          frame False {
          }
          frame True {
            n283 = call "规范时间戳.vi"("字符串"=w518) -> ("result string"=w520:string)  [unwired: 10 in]
            n284 = Format Into String(format string="DataTime=%s;%s", w520, w517) -> (resulting string=w516:string)  [unwired: 2 in, 1 out]
          }
        }
      }
    }
  }
  "字符串" <- w11
